vi "Cache.FindOldFiles.vi"(7 "Idx":i32, 8 "error in":errorcluster, 11 "Data in":T1) -> (0 "error out":errorcluster, 1 "Found?":bool, 2 "files to remove":path[](array[path]), 3 "Data out":T1)   [LabVIEW 2016]
uses:
  Cache.Data.ctl
  Cache.Data.Status.ctl
  Cache.Data.Sets.ctl
  Global/ApplicationGlobal.vi
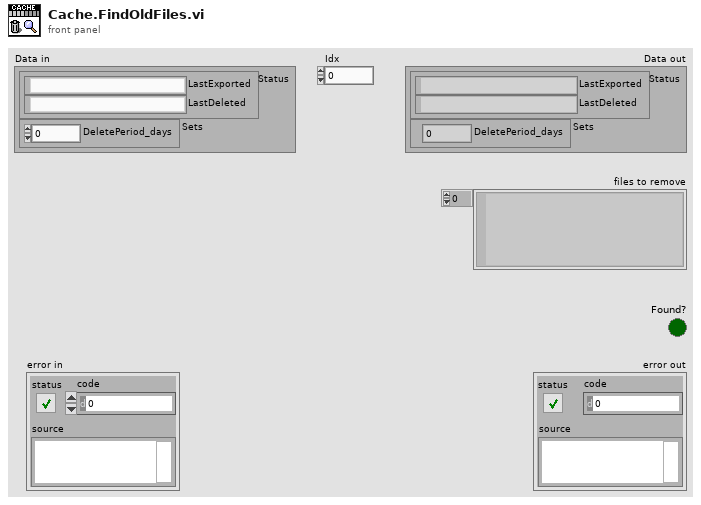
[diagram p1: front panel]
types:
  T1 = typedef "Cache.Data.ctl" = cluster{"Status":T2, "Sets":T3}
  T2 = typedef "Cache.Data.Status.ctl" = cluster{"LastExported":string, "LastDeleted":string}
  T3 = typedef "Cache.Data.Sets.ctl" = cluster{"DeletePeriod_days":dbl}
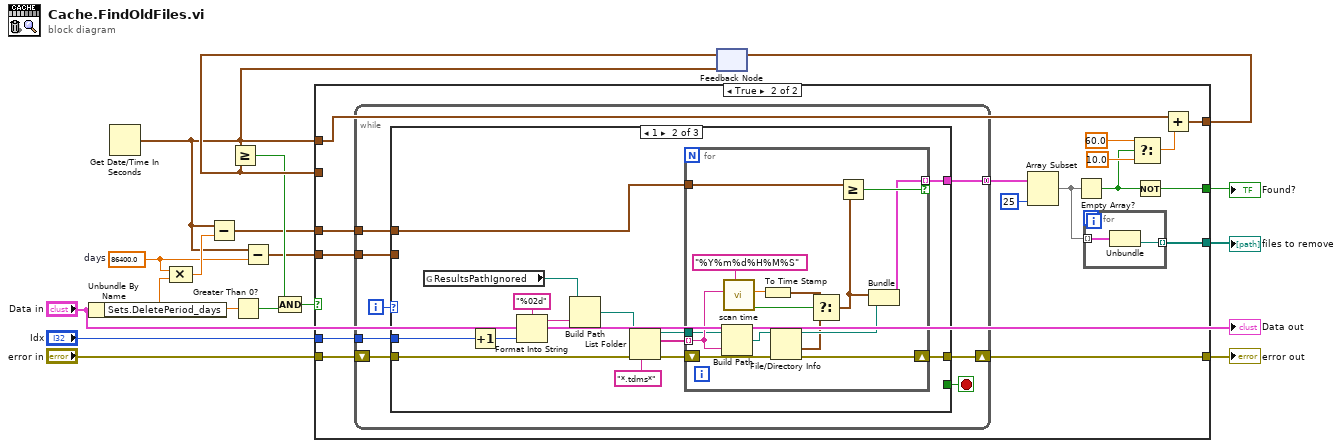
[diagram p0: block diagram]
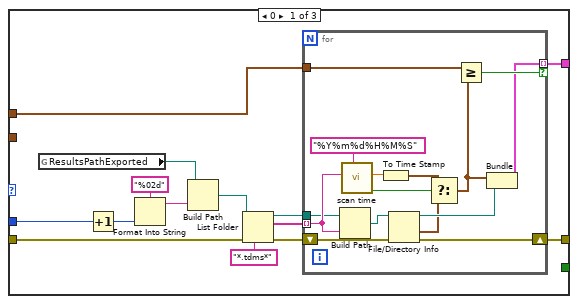
[diagram p3: hidden frame]
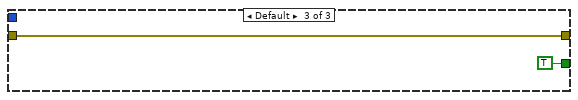
[diagram p4: hidden frame]
diagram:
  w3 = 86400.0  # days
  n1 = Unbundle By Name("Data in") -> ("Sets.DeletePeriod_days"=w4:dbl)
  n2 = Get Date/Time In Seconds() -> (seconds since 1Jan1904=w8:timestamp)
  n3 = Compound Arithmetic op=MULTIPLY(w3, w4) -> (w11:dbl)
  n4 = Subtract(x=w8, y=w11) -> (x-y=w10:timestamp)
  n5 = Greater Than 0?(x=w4) -> (x > 0?=w5:bool)
  n6 = Subtract(x=w8, y=w3) -> (x-y=w7:timestamp)
  n7 = feedback #1(w8) -> (w15:timestamp)
  n8 = Greater Or Equal?(x=w8, y=w15) -> (x >= y?=w12:bool)
  n9 = Compound Arithmetic op=AND(w12, w5) -> (w13:bool)
  n10 = case shown="True" w13 {
    tunnel: "error in" -> [w18 w35]
    tunnel: w8 -> [_ w26]
    tunnel: [w19 w33] -> w16
    tunnel: w15 -> [w19 _]
    tunnel: [w18 w24] -> w14
    tunnel: [_ w29] -> w9
    tunnel: w10 -> [_ w31]
    tunnel: w7 -> [_ w27]
    tunnel: "Idx" -> [_ w25]
    tunnel: [_ w20] -> w2
    frame False {
    }
    frame True {
      n11 = while {
        tunnel: [w42] -> w23 mode=concatenating
        shift-right: [w41] -> w24
        shift-left: w35 -> [w43]
        tunnel: w31 -> [w38]
        tunnel: w27 -> [w37]
        tunnel: w25 -> [w36]
        i -> [w40]
        stop <- w39 stop-if-true
        n12 = case shown="1" w40 {
          tunnel: w43 -> [w57 w86 w102]
          tunnel: [w54 w83 _] -> w42
          tunnel: [w52 w81 w102] -> w41
          tunnel: [_ _ TRUE] -> w39
          tunnel: w38 -> [w50 w79 _]
          tunnel: w37 -> [_ _ _]
          tunnel: w36 -> [w46 w75 _]
          frame 0 {
            n13 = global read "ApplicationGlobal.vi" "ResultsPathExported"() -> (w49:path)
            n14 = Increment(x=w46) -> (x+1=w47:i32)
            n15 = Format Into String(format string="%02d", w47) -> (resulting string=w45:string)  [unwired: 2 in, 1 out]
            n16 = Build Path(base path=w49, name or relative path=w45) -> (appended path=w44:path)
            n17 = List Folder(path=w44, pattern="*.tdms*", error in=w57) -> (path out=w51:path, filenames=w56:string[], error out=w55:errorcluster)  [unwired: 1 in, 1 out]
            n18 = for {
              tunnel: w56 -> [w65] mode=indexing
              tunnel: w51 -> [w64]
              shift-right: [w71] -> w52
              shift-left: w55 -> [w72]
              tunnel: w50 -> [w70]
              tunnel: [w67] -> w54 mode=indexing if=w69
              n19 = Build Path(base path=w64, name or relative path=w65) -> (appended path=w68:path)
              n20 = call "scan time.vi"("time format string"="%Y%m%d%H%M%S", "formatted time string"=w65) -> ("ok?"=w61:bool, "lv time (UTC)"=w62:dbl)  [unwired: 5 in, 3 out]
              n21 = To Time Stamp(1:w62) -> (0:w60:timestamp)
              n22 = File/Directory Info(path=w68, error in=w72) -> (path out=w66:path, last mod=w59:timestamp, error out=w71:errorcluster)  [unwired: 4 out]
              n23 = Select(t=w60, s=w61, f=w59) -> (s? t:f=w58:timestamp)
              n24 = Greater Or Equal?(x=w70, y=w58) -> (x >= y?=w69:bool)
              n25 = Bundle("last mod"=w58, "path out"=w66) -> (w67:cluster{"last mod":timestamp, "path out":path})  [unwired: 1 in]
            }
          }
          frame 1 {
            n26 = global read "ApplicationGlobal.vi" "ResultsPathIgnored"() -> (w78:path)
            n27 = Increment(x=w75) -> (x+1=w76:i32)
            n28 = Format Into String(format string="%02d", w76) -> (resulting string=w74:string)  [unwired: 2 in, 1 out]
            n29 = Build Path(base path=w78, name or relative path=w74) -> (appended path=w73:path)
            n30 = List Folder(path=w73, pattern="*.tdms*", error in=w86) -> (path out=w80:path, filenames=w85:string[], error out=w84:errorcluster)  [unwired: 1 in, 1 out]
            n31 = for {
              tunnel: w85 -> [w94] mode=indexing
              tunnel: w80 -> [w93]
              shift-right: [w100] -> w81
              shift-left: w84 -> [w101]
              tunnel: w79 -> [w99]
              tunnel: [w96] -> w83 mode=indexing if=w98
              n32 = Build Path(base path=w93, name or relative path=w94) -> (appended path=w97:path)
              n33 = call "scan time.vi"("time format string"="%Y%m%d%H%M%S", "formatted time string"=w94) -> ("ok?"=w90:bool, "lv time (UTC)"=w91:dbl)  [unwired: 5 in, 3 out]
              n34 = To Time Stamp(1:w91) -> (0:w89:timestamp)
              n35 = File/Directory Info(path=w97, error in=w101) -> (path out=w95:path, last mod=w88:timestamp, error out=w100:errorcluster)  [unwired: 4 out]
              n36 = Select(t=w89, s=w90, f=w88) -> (s? t:f=w87:timestamp)
              n37 = Greater Or Equal?(x=w99, y=w87) -> (x >= y?=w98:bool)
              n38 = Bundle("last mod"=w87, "path out"=w95) -> (w96:cluster{"last mod":timestamp, "path out":path})  [unwired: 1 in]
            }
          }
          frame Default {
          }
        }
      }
      n39 = Array Subset(array=w23, length=25) -> (w28:cluster{"last mod":timestamp, "path out":path}[])  [unwired: 1 in]
      n40 = Empty Array?(array=w28) -> (empty?=w21:bool)
      n41 = for {
        tunnel: w28 -> [w105] mode=indexing
        tunnel: [w104] -> w29 mode=indexing
        n42 = Unbundle(w105) -> ("path out"=w104:path)  [unwired: 1 out]
      }
      n43 = Select(t=60.0 ("x"), s=w21, f=10.0) -> (s? t:f=w34:dbl)
      n44 = Not(x=w21) -> (.not. x?=w20:bool)
      n45 = Add(x=w26, y=w34) -> (x+y=w33:timestamp)
    }
  }
  "error out" <- w14
  "files to remove" <- w9
  "Found?" <- w2
  n46 = feedback-in #1(w16) -> ()
  "Data out" <- "Data in"
